vi "Simulated Elevator.vi"(9 "Top":bool, 10 "Middle":bool, 11 "Bottom":bool) -> (3 "in Range":bool)   [LabVIEW 2014]
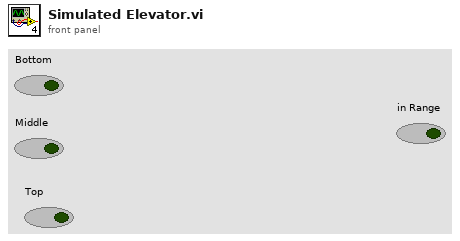
[diagram p1: front panel]
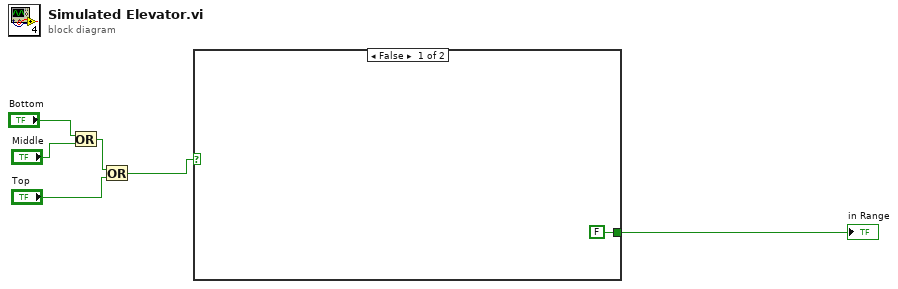
[diagram p0: block diagram]
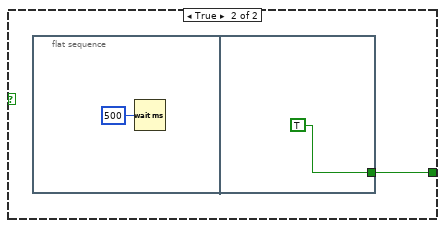
[diagram p2: hidden frame]
diagram:
  n1 = Or(x="Bottom", y="Middle") -> (x .or. y?=w6:bool)
  n2 = Or(x=w6, y="Top") -> (x .or. y?=w5:bool)
  n3 = case shown="False" w5 {
    tunnel: [FALSE w8] -> w1
    frame False {
    }
    frame True {
      n4 = flat-sequence {
        tunnel: [TRUE] -> w8
        frame #0 {
          n5 = Wait (ms)(milliseconds to wait=u32 500) -> ()  [unwired: 1 out]
        }
        frame #1 {
        }
      }
    }
  }
  "in Range" <- w1
